vi "Default Labels.vi"(8 "error in (no error)":errorcluster, 11 "PieChart in":refnum<class "PieChart.lvclass">) -> (0 "error out":errorcluster, 3 "PieChart out":refnum<class "PieChart.lvclass">)   [LabVIEW 2020, in "PieChart.lvclass"]
uses:
  PieChart.lvclass
  PieChart.lvclass/PieChart.ctl
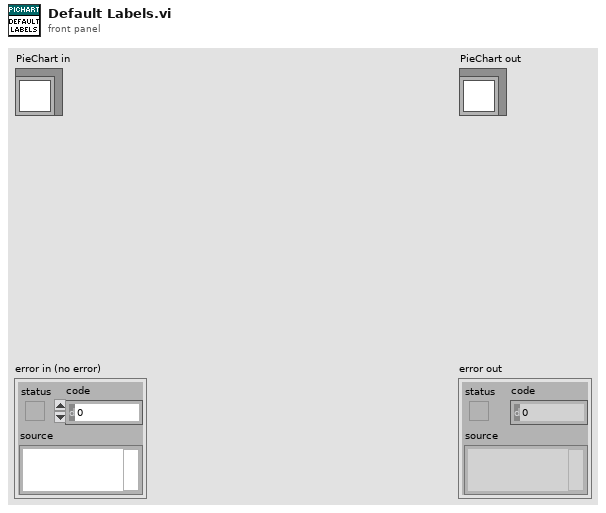
[diagram p1: front panel]
types:
  T1 = typedef "PieChart.lvclass/State Data.ctl" = cluster{"Title":string, "Values[]":dbl[], "Labels[]":string[], "Colors[]":u32[], "Include Legend?":bool, "Include Title?":bool, "Title Font":T2, "Legend Font":T2, "Selection":i32, "Slice Positions":T3}
  T2 = typedef "LVFontTypeDef.ctl" = cluster{"Font Name":string, "Size":u16, "Bold":bool, "Italic":bool, "Underline":bool, "Strikeout":bool, "Color":u32}
  T3 = typedef "PieChart.lvclass/Pie info for Click.ctl" = cluster{"Slice Positions":cluster{"Start":i16, "End":i16}[], "Center Position":T4, "Radius":i16}
  T4 = typedef "LVBoundsTypeDef.ctl" = cluster{"Width":u32, "Height":u32}
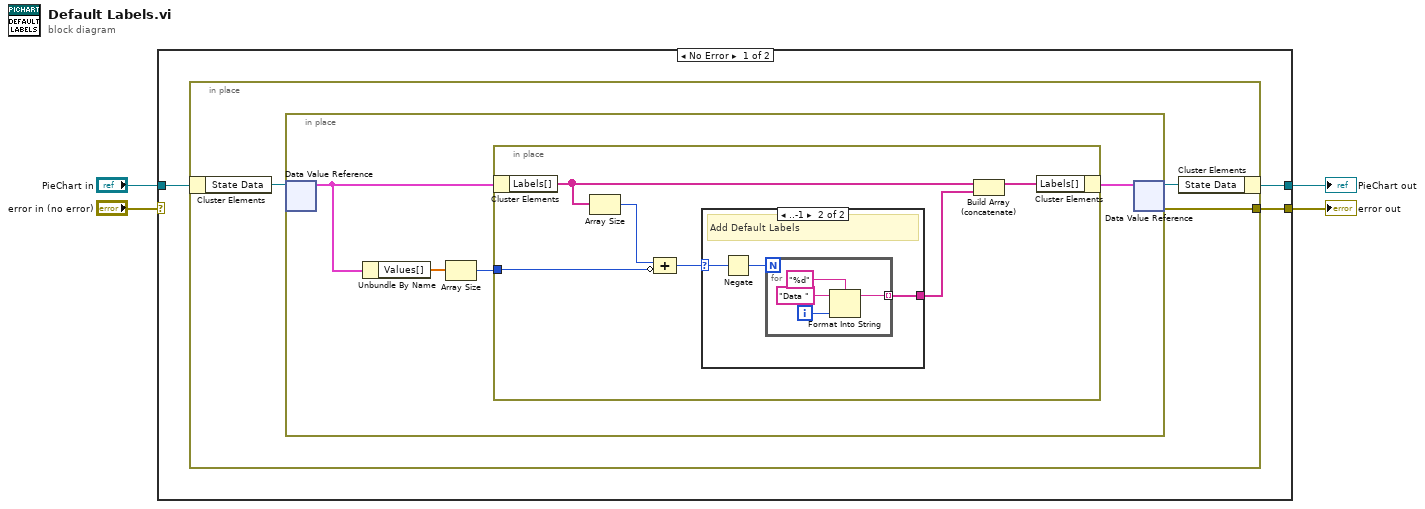
[diagram p0: block diagram]
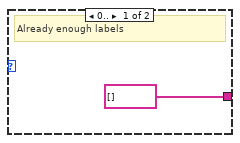
[diagram p2: hidden frame]
diagram:
  n1 = case shown="No Error" "error in (no error)" {
    selector: "error in (no error)" -> [_ w30]
    tunnel: [w6 w30] -> w3
    tunnel: [w5 w29] -> w1
    tunnel: "PieChart in" -> [w7 w29]
    frame No Error {
      n2 = in-place {
        in-place-border: [w8] -> w6
        n3 = in-place-cluster #1(w7) -> ("State Data"=w10:refnum<data-value>)
        n4 = in-place {
          n5 = in-place-dvr #2(w10) -> (w14:T1)  [unwired: 1 out]
          n6 = Unbundle By Name(w14) -> ("Values[]"=w12:dbl[])
          n7 = Array Size(array=w12) -> (size(s)=w11:i32)
          n8 = in-place {
            in-place-border: w11 -> [w19]
            n9 = in-place-cluster #3(w14) -> ("Labels[]"=w18:string[])
            n10 = Array Size(array=w18) -> (size(s)=w20:i32)
            n11 = Compound Arithmetic op=ADD(w20, invert w19) -> (w16:i32)
            n12 = case shown="..-1" w16 {
              selector: w16 -> [_ w24]
              tunnel: [string[] [] ("array") w23] -> w15
              frame 0.. {
                # "Already enough labels"
              }
              frame ..-1 {
                # "Add Default Labels"
                n13 = Negate(x=w24) -> (-x=w22:i32)
                n14 = for {
                  N: w22 -> [_]
                  tunnel: [w25] -> w23 mode=indexing
                  i -> [w28]
                  n15 = Format Into String(format string="%d", initial string="Data ", w28) -> (resulting string=w25:string)  [unwired: 1 in, 1 out]
                }
              }
            }
            n16 = Build Array (concatenate)(w18, w15) -> (w17:string[])
            n17 = in-place-cluster #3("Labels[]"=w17) -> (w13:T1)
          }
          n18 = in-place-dvr #2(w13) -> (w9:refnum<data-value>, w8:errorcluster)
        }
        n19 = in-place-cluster #1("State Data"=w9) -> (w5:refnum<class "PieChart.lvclass">)
      }
    }
    frame Error {
    }
  }
  "error out" <- w3
  "PieChart out" <- w1
